vi "SyncedRec_sub.vi"(0 "minimum value":dbl=-10.0 caption="Output Minimum Value" format="%0.2f", 1 "signal in":waveform(dbl), 2 "rate":dbl=500000.0 caption="Update Generation Rate" format="%0.2f", 3 "Samples to Read":i32=262144, 5 "maximum value":dbl=10.0 caption="Output Maximum Value" format="%0.2f", 7 "Physical Channel":tag="Dev1/ai0" caption="Input Physical Channel", 9 "physical channels":tag="Dev1/ao0" caption="Output Physical Channels", 11 "Rate":dbl=500000.0 caption="Input Rate" format="%0.2f", 12 "Analog Input Sample Clock Source":tag="/Dev1/ao/SampleClock", 13 "Minimum Value":dbl=-10.0 caption="Input Minimum Value" format="%0.2f", 14 "Maximum Value":dbl=10.0 caption="Input Maximum Value" format="%0.2f") -> (4 "Actual Input Rate":dbl=10000.0 format="%0.2f", 6 "data":waveform(dbl), 8 "Actual Update Generation Rate":dbl=5000.0 format="%0.2f")   [LabVIEW 2017]
uses:
  <vilib>/Utility/error.llb/DialogType.ctl
  <vilib>/DAQmx/write.llb/DAQmx Write (Analog Wfm 1Chan NSamp).vi
  <vilib>/DAQmx/read.llb/DAQmx Read (Analog Wfm 1Chan NSamp).vi
  <vilib>/DAQmx/create/channels.llb/DAQmx Create Channel (AO-Voltage-Basic).vi
  <vilib>/DAQmx/configure/timing.llb/DAQmx Timing (Sample Clock).vi
  <vilib>/DAQmx/miscellaneous.llb/DAQmx Fill In Error Info.vi
  <vilib>/DAQmx/create/channels.llb/DAQmx Create Channel (AI-Voltage-Basic).vi
  <vilib>/DAQmx/configure/trigger.llb/DAQmx Start Trigger (Digital Edge).vi
  <resource>/objmgr/daqmx.rc
panel:
  in  "Analog Input Trigger Source":tag="/Dev1/ao/StartTrigger"
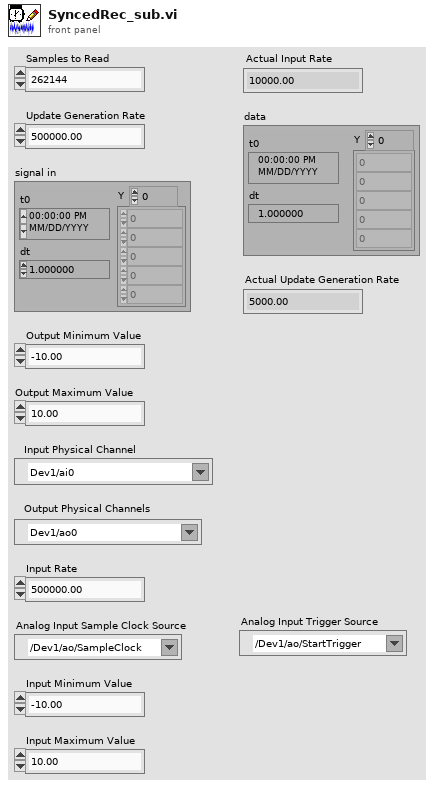
[diagram p1: front panel]
types:
  T1 = typedef "DialogType.ctl" = u16
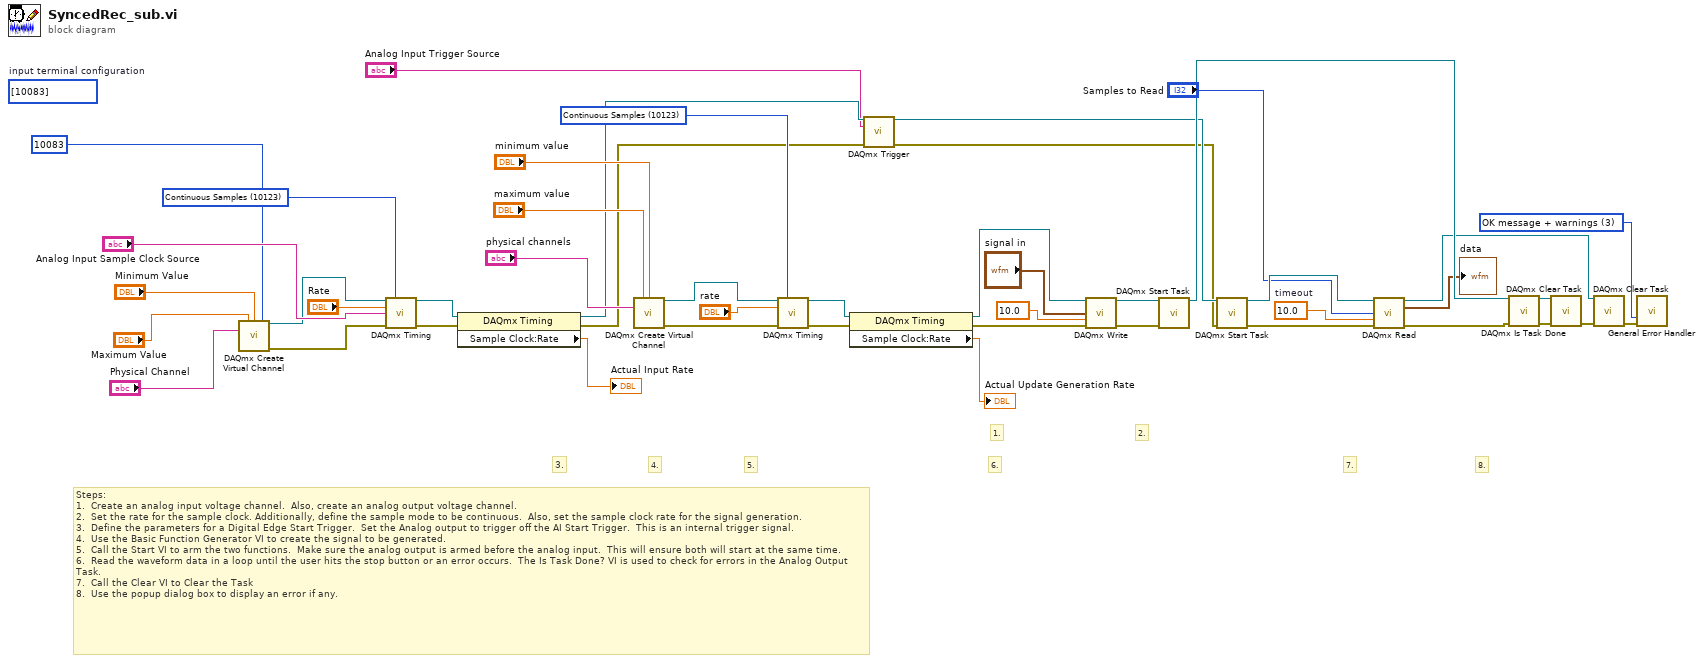
[diagram p0: block diagram]
diagram:
  (unwired) i32[] [10083] items=["default"=-1, "RSE"=10083, "NRSE"=10078, "Differential"=10106, "Pseudodifferential"=12529]  # input terminal configuration
  w38 = 10.0  # timeout
  w23 = T1 3 items=["no dialog", "OK message", "continue or stop message", "OK message + warnings", "continue/stop + warnings"] ("type of dialog (OK msg:1)")
  w15 = 10123 items=["Finite Samples"=10178, "Continuous Samples"=10123] ("sample mode")
  w9 = 10123 items=["Finite Samples"=10178, "Continuous Samples"=10123] ("sample mode")
  # "6."
  # "3."
  # "4."
  # "8."
  # "5."
  # "7."
  # "Steps: \n1.  Create an analog input voltage channel.  Also, create an analog output voltage channel.\n2.  Set the rate for the sample clock. Additionally, define the sample mode to be continuous.  Also, set the sample clock rate for the signal generation.\n3.  Define the parameters for a Digital Edge Start Trigger.  Set the Analog output to trigger off the AI Start Trigger.  This is an internal trigger signal.\n4.  Use the Basic Function Generator VI to create the signal to be generated.\n5.  Call the Start VI to arm the two functions.  Make sure the analog output is armed before the analog input.  This will ensure both will start at the same time.\n6.  Read the waveform data in a loop until the user hits the stop button or an error occurs.  The Is Task Done? VI is used to check for errors in the Analog Output Task.\n7.  Call the Clear VI to Clear the Task\n8.  Use the popup dialog box to display an error if any."
  # "2."
  # "1."
  n1 = call-poly <vilib>:"DAQmx Create Virtual Channel.vi"("maximum value"="Maximum Value", "minimum value"="Minimum Value", "input terminal configuration"=10083, "physical channels"="Physical Channel") -> ("task out"=w11:refnum<k21>, "error out"=w10:errorcluster)  [unwired: 10 in]
  n2 = call-poly <vilib>:"DAQmx Timing.vi"("task/channels in"=w11, "sample mode"=w9, "rate"="Rate", "source"="Analog Input Sample Clock Source", "error in"=w10) -> ("task out"=w28:refnum<k21>, "error out"=w29:errorcluster)  [unwired: 9 in]
  n3 = property class="DAQmx Timing"(reference=w28, error in=w29) -> (reference out=w4:refnum<k21>, error out=w5:errorcluster, "Sample Clock:Rate"=→"Actual Input Rate":dbl)
  n4 = call-poly <vilib>:"DAQmx Create Virtual Channel.vi"("maximum value"="maximum value", "minimum value"="minimum value", "physical channels"="physical channels") -> ("task out"=w16:refnum<k21>, "error out"=w17:errorcluster)  [unwired: 11 in]
  n5 = call-poly <vilib>:"DAQmx Timing.vi"("task/channels in"=w16, "sample mode"=w15, "rate"="rate", "error in"=w17) -> ("task out"=w25:refnum<k21>, "error out"=w26:errorcluster)  [unwired: 10 in]
  n6 = property class="DAQmx Timing"(reference=w25, error in=w26) -> (reference out=w33:refnum<k21>, error out=w34:errorcluster, "Sample Clock:Rate"=→"Actual Update Generation Rate":dbl)
  n7 = call-poly <vilib>:"DAQmx Trigger.vi"("task/channels in"=w4, "source"="Analog Input Trigger Source", "error in"=w5) -> ("task out"=w2:refnum<k21>, "error out"=w1:errorcluster)  [unwired: 11 in]
  n8 = call-poly <vilib>:"DAQmx Write.vi"("task/channels in"=w33, "data"="signal in", "timeout"=10.0 ("Wirite Timeout"), "error in"=w34) -> ("task out"=w20:refnum<k21>, "error out"=w21:errorcluster)  [unwired: 9 in, 1 out]
  n9 = call <vilib>:"DAQmx Start Task.vi"("task/channels in"=w20, "error in"=w21) -> ("task out"=w43:refnum<k21>)  [unwired: 12 in, 1 out]
  n10 = call <vilib>:"DAQmx Start Task.vi"("task/channels in"=w2, "error in"=w1) -> ("task out"=w41:refnum<k21>, "error out"=w42:errorcluster)  [unwired: 12 in]
  n11 = call-poly <vilib>:"DAQmx Read.vi"("task/channels in"=w41, "number of samples per channel"="Samples to Read", "timeout"=w38, "error in"=w42) -> ("task out"=w40:refnum<k21>, "data"=→"data":waveform(dbl), "error out"=w36:errorcluster)  [unwired: 9 in]
  n12 = call <vilib>:"DAQmx Is Task Done.vi"("task/channels in"=w43, "error in"=w36) -> ("task out"=w45:refnum<k21>, "error out"=w44:errorcluster)  [unwired: 11 in, 1 out]
  n13 = call <vilib>:"DAQmx Clear Task.vi"("task in"=w45, "error in"=w44) -> ("error out"=w31:errorcluster)  [unwired: 13 in]
  n14 = call <vilib>:"DAQmx Clear Task.vi"("task in"=w40, "error in"=w31) -> ("error out"=w32:errorcluster)  [unwired: 13 in]
  n15 = call <vilib>:"General Error Handler.vi"("type of dialog (OK msg:1)"=w23, "error in (no error)"=w32) -> ()  [unwired: 9 in, 5 out]
